vi "getXMLPoint.vi"(11 "Point Node":refnum<k20>) -> (1 "y":dbl, 3 "x":dbl)   [LabVIEW 2013]
doc: "This vi extracts the coordinates x and y from a xml <B>Point</B> node"
uses:
  <vilib>/xml/NI_XML.lvlib
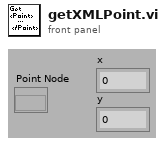
[diagram p1: front panel]
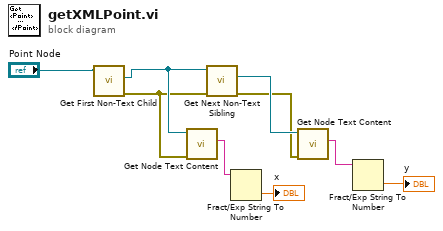
[diagram p0: block diagram]
diagram:
  n1 = call <vilib>:"Get First Non-Text Child.vi"("node in"="Point Node") -> ("error out"=w3:errorcluster, "child node"=w4:refnum<k20>)  [unwired: 7 in, 2 out]
  n2 = call <vilib>:"Get Node Text Content.vi"("error in (no error)"=w3, "node in"=w4) -> ("node text"=w9:string)  [unwired: 7 in, 2 out]
  n3 = call <vilib>:"Get Next Non-Text Sibling.vi"("error in (no error)"=w3, "node in"=w4) -> ("error out"=w1:errorcluster, "sibling node"=w2:refnum<k20>)  [unwired: 6 in, 2 out]
  n4 = Fract/Exp String To Number(string=w9) -> (number=→"x":dbl)  [unwired: 3 in, 1 out]
  n5 = call <vilib>:"Get Node Text Content.vi"("error in (no error)"=w1, "node in"=w2) -> ("node text"=w8:string)  [unwired: 7 in, 2 out]
  n6 = Fract/Exp String To Number(string=w8) -> (number=→"y":dbl)  [unwired: 3 in, 1 out]
